vi "reset_written_status.vi"(8 "error in (no error)":errorcluster, 11 "DAQmxWriteSignals in":refnum<class "SignalWriterMM140725DAQmx.lvclass">) -> (0 "error out":errorcluster, 3 "DAQmxWriteSignals out":refnum<class "SignalWriterMM140725DAQmx.lvclass">)   [LabVIEW 2010, in "SignalWriterMM140725DAQmx.lvclass"]
uses:
  SignalWriterMM140725DAQmx.lvclass
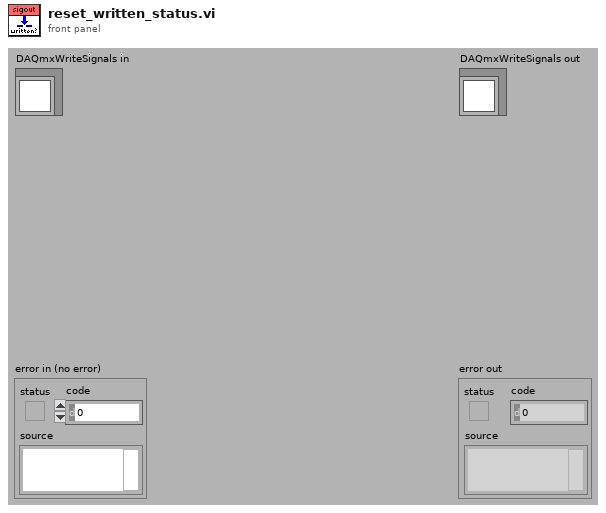
[diagram p1: front panel]
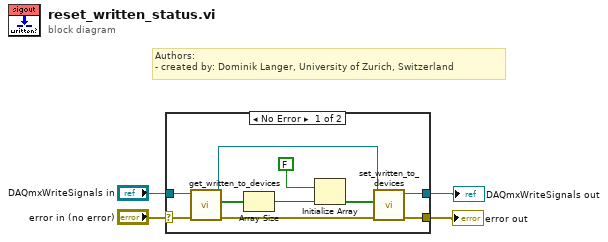
[diagram p0: block diagram]
diagram:
  # "Authors: \n- created by: Dominik Langer, University of Zurich, Switzerland"
  n1 = case shown="No Error" "error in (no error)" {
    selector: "error in (no error)" -> [w14 w16]
    tunnel: [w8 w16] -> w3
    tunnel: [w6 w15] -> w1
    tunnel: "DAQmxWriteSignals in" -> [w13 w15]
    frame No Error {
      n2 = call-dynamic "get_written_to_devices.vi"("error in (no error)"=w14, "DAQmxWriteSignals in"=w13) -> ("error out"=w9:errorcluster, "written to devices?"=w12:bool[], "DAQmxWriteSignals out"=w5:refnum<class "SignalWriterMM140725DAQmx.lvclass">)  [unwired: 7 out]
      n3 = Array Size(array=w12) -> (size(s)=w11:i32)
      n4 = Initialize Array(FALSE, w11) -> (w7:bool[])
      n5 = call-dynamic "set_written_to_devices.vi"("error in (no error)"=w9, "written to devices?"=w7, "DAQmxWriteSignals in"=w5) -> ("error out"=w8:errorcluster, "DAQmxWriteSignals out"=w6:refnum<class "SignalWriterMM140725DAQmx.lvclass">)  [unwired: 7 out]
    }
    frame Error {
    }
  }
  "error out" <- w3
  "DAQmxWriteSignals out" <- w1
